vi "Robot Arm Control.vi"(8 "Rate Control K":dbl, 9 "Home y":dbl=36.0 format="%#_13g", 10 "Home x":dbl=3.5 format="%#_13g", 11 "Desired Coordinates":cluster{"x":dbl, "y":dbl}) -> (0 "Arm at point":bool)   [LabVIEW 2015]
uses:
  Sensors.vi
panel:
  out "Current X":dbl
  out "Current Y":dbl
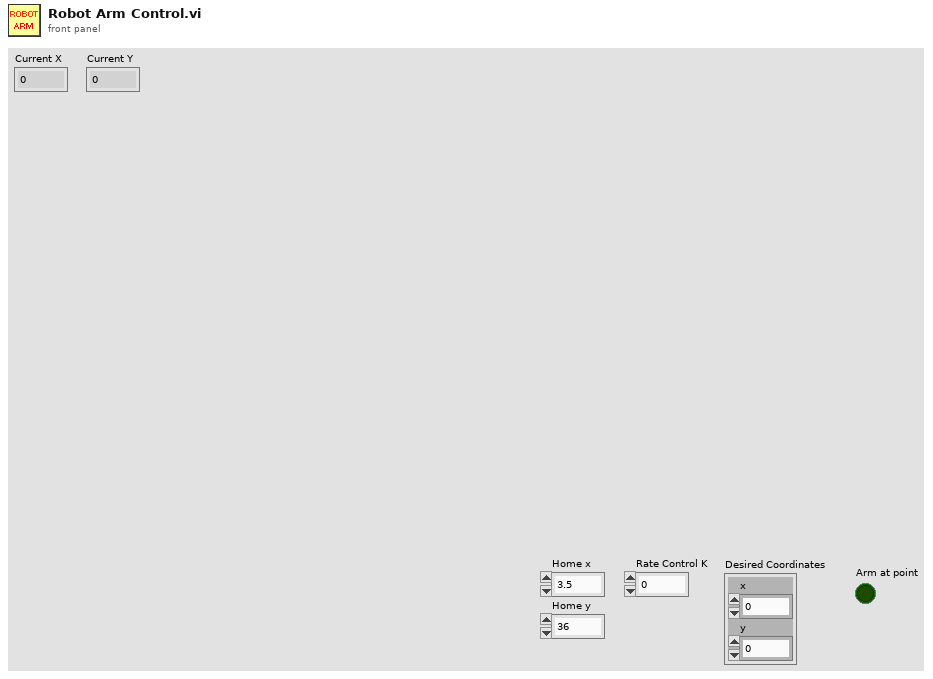
[diagram p1: front panel]
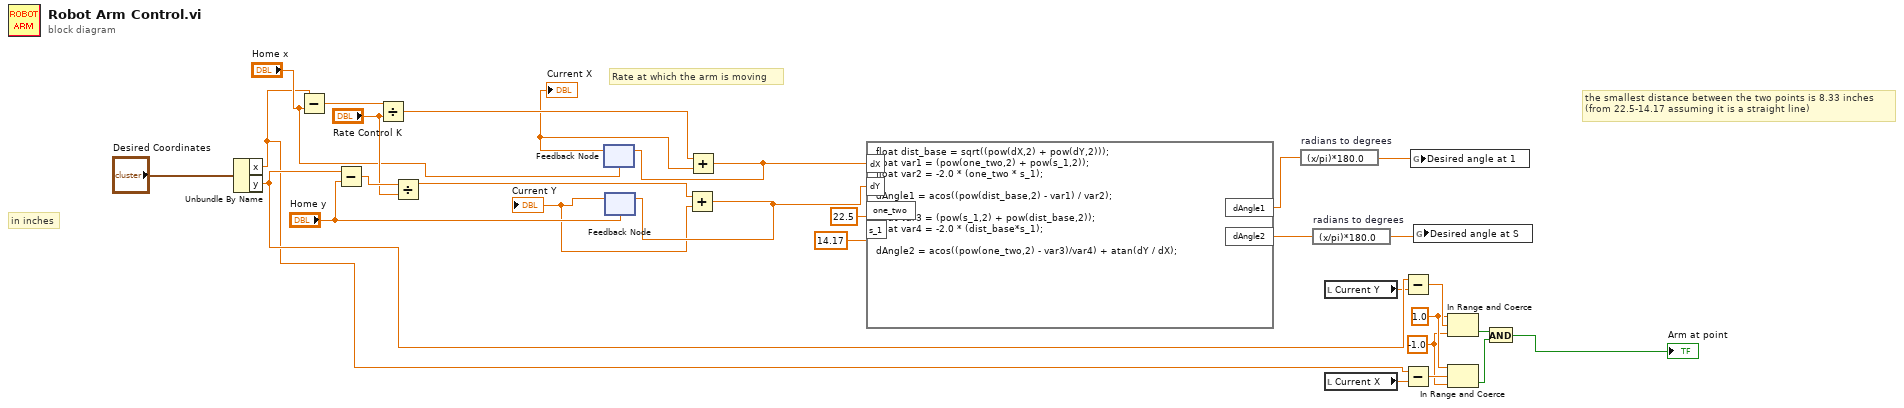
[diagram p0: block diagram]
diagram:
  w5 = -1.0 ("upper limit")
  w6 = 1.0 ("upper limit")
  # "Rate at which the arm is moving"
  # "the smallest distance between the two points is 8.33 inches\n(from 22.5-14.17 assuming it is a straight line)"
  # "in inches"
  n1 = Unbundle By Name("Desired Coordinates") -> ("x"=w20:dbl, "y"=w21:dbl)
  n2 = Subtract(x=w20, y="Home x") -> (x-y=w28:dbl)
  n3 = Subtract(x=w21, y="Home y") -> (x-y=w27:dbl)
  n4 = Divide(x=w28, y="Rate Control K") -> (x/y=w22:dbl)
  n5 = Divide(x=w27, y="Rate Control K") -> (x/y=w23:dbl)
  n6 = feedback #1("Home x") -> (w16:dbl)
  "Current X" <- w16
  n7 = feedback #2("Home y") -> (w11:dbl)
  "Current Y" <- w11
  n8 = Add(x=w23, y=w11) -> (x+y=w14:dbl)
  n9 = feedback-in #2(w14) -> ()
  n10 = Add(x=w22, y=w16) -> (x+y=w15:dbl)
  n11 = feedback-in #1(w15) -> ()
  n12 = formula code="float dist_base = sqrt((pow(dX,2) + pow(dY,2)));\nfloat var1 = (pow(one_two,2) + pow(s_1,2));\nfloat var2 = -2.0 * (one_two * s_1);\n\ndAngle1 = acos((pow(dist_base,2) - var1) / var2);\n\nfloat var3 = (pow(s_1,2) + pow(dist_base,2));\nfloat var4 = -2.0 * (dist_base*s_1);\n\ndAngle2 = acos((pow(one_two,2) - var3)/var4) + atan(dY / dX);"("dX"=w15, "dY"=w14, "one_two"=22.5 ("input variable"), "s_1"=14.17 ("input variable")) -> ("dAngle1"=w18:dbl, "dAngle2"=w17:dbl)
  n13 = expression code="(x/pi)*180.0" "radians to degrees"(w18) -> (w2:dbl)
  n14 = expression code="(x/pi)*180.0" "radians to degrees"(w17) -> (w1:dbl)
  n15 = local read "Current Y"() -> (w10:dbl)
  n16 = local read "Current X"() -> (w8:dbl)
  n17 = Subtract(x=w21, y=w10) -> (x-y=w9:dbl)
  n18 = Subtract(x=w20, y=w8) -> (x-y=w7:dbl)
  n19 = global write "Sensors.vi" "Desired angle at 1"(w2) -> ()
  n20 = global write "Sensors.vi" "Desired angle at S"(w1) -> ()
  n21 = In Range and Coerce(upper limit=w6, x=w9, lower limit=w5) -> (In Range?=w4:bool)  [unwired: 1 out]
  n22 = In Range and Coerce(upper limit=w6, x=w7, lower limit=w5) -> (In Range?=w3:bool)  [unwired: 1 out]
  n23 = And(x=w4, y=w3) -> (x .and. y?=→"Arm at point":bool)
